vi "gen rand secenario.vi"(8 "error in (no error)":errorcluster, 10 "rand limits":T3={"# Number of emitters"=84, "# Number of frequency per emitter"={"Numeric"=0, "Numeric"=22}, "Frequency range"={"Numeric"=158778625.95419848, "Numeric"=2894656488.5496182}, "Frequency dispersion for each emitter"={"Numeric"=0.0, "Numeric"=1181732.2396298076}, "PRF range (Hz)"={"Numeric"=33.59056776941936, "Numeric"=576.0533087800792}, "Duty cycle - pulse in PRI"={"Numeric"=0.026717557251908396, "Numeric"=0.11832061068702289}, "Amplitude (dB)"={"Numeric"=-34.62595419847328, "Numeric"=-51.11450381679389}, "Modulation depth"={"Numeric"=19162.08437325717, "Numeric"=1181732.2396298076}, "CW"=TRUE, "LFM"=TRUE, "DOA (DEG)"={"Numeric"=0.0, "Numeric"=1181732.2396298076}, "start time (Sec)"=0.0, "end time (Sec)"=50.0, "BPSK"=TRUE, "QPSK"=TRUE, "ARB"=FALSE} {"DOA (DEG)" scale=0.0..360.0 scale format="%#_6f"; "Modulation depth" scale=1000.0..10000000.0 scale format="%#_6pHz"; "Amplitude (dB)" scale format="%#_6fdB"; "Duty cycle - pulse in PRI" scale=0.0..1.0 scale format="%#_6f"; "PRF range (Hz)" scale=1.0..3000.0 scale format="%#_6pHz"; "Frequency dispersion for each emitter" scale=1000000.0..100000000.0 scale format="%#_6pHz"; "Frequency range" scale=975000000.0..2225000000.0 scale format="%#_4pHz"; "# Number of frequency per emitter" scale=0.01..3000.0; "# Number of emitters" scale=0.0..200.0}, 11 "device_type in":refnum<class "device_type.lvclass">) -> (0 "error out":errorcluster, 2 "transmitters":T1[](array[typedef]) {"t end" format="%#_3p"; "t start" format="%#_3p"; "DOA" format="%#_3p"; "mod depth" format="%#_3p"}, 3 "device_type out":refnum<class "device_type.lvclass">)   [LabVIEW 2021, in "device_type.lvclass"]
uses:
  device_type.lvclass
  pulse_tx_vis/CTL/random_limits.ctl
  pulse_tx_vis/CTL/emitter params.ctl
  pulse_tx_vis/CTL/mode_type.ctl
  <vilib>/numeric/Random Number (Range) DBL.vi
  <vilib>/numeric/Random Number (Range) U64.vi
  <vilib>/numeric/sub_Random U32.vi
  device_type.lvclass/device_type.ctl
panel:
  # "modulation \ntypes:"
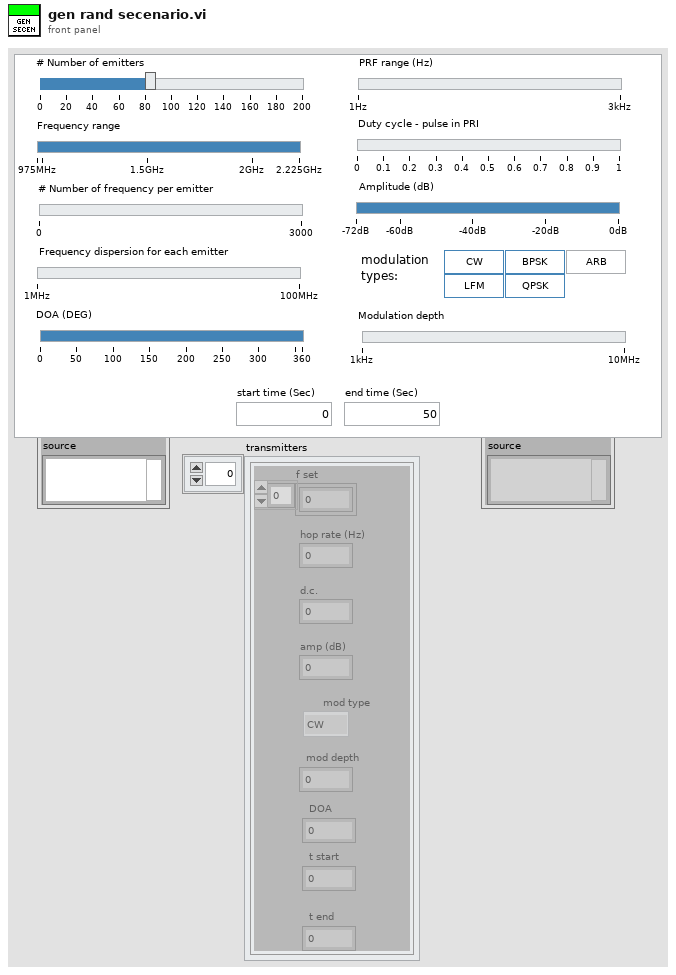
[diagram p1: front panel]
types:
  T1 = typedef "emitter params.ctl" = cluster{"f set":dbl[], "hop rate (Hz)":dbl, "d.c.":dbl, "amp (dB)":dbl, "mod type":T2, "mod depth":dbl, "DOA":dbl, "t start":dbl, "t end":dbl}
  T2 = typedef "mode_type.ctl" = enum8{"CW", "from memory 1", "NC - cw", "LFM", "BPSK", "QPSK"}
  T3 = typedef "random_limits.ctl" = cluster{"# Number of emitters":u32, "# Number of frequency per emitter":cluster{"Numeric":u32, "Numeric":u32}, "Frequency range":cluster{"Numeric":dbl, "Numeric":dbl}, "Frequency dispersion for each emitter":cluster{"Numeric":dbl, "Numeric":dbl}, "PRF range (Hz)":cluster{"Numeric":dbl, "Numeric":dbl}, "Duty cycle - pulse in PRI":cluster{"Numeric":dbl, "Numeric":dbl}, "Amplitude (dB)":cluster{"Numeric":dbl, "Numeric":dbl}, "Modulation depth":cluster{"Numeric":dbl, "Numeric":dbl}, "CW":bool, "LFM":bool, "DOA (DEG)":cluster{"Numeric":dbl, "Numeric":dbl}, "start time (Sec)":dbl, "end time (Sec)":dbl, "BPSK":bool, "QPSK":bool, "ARB":bool}
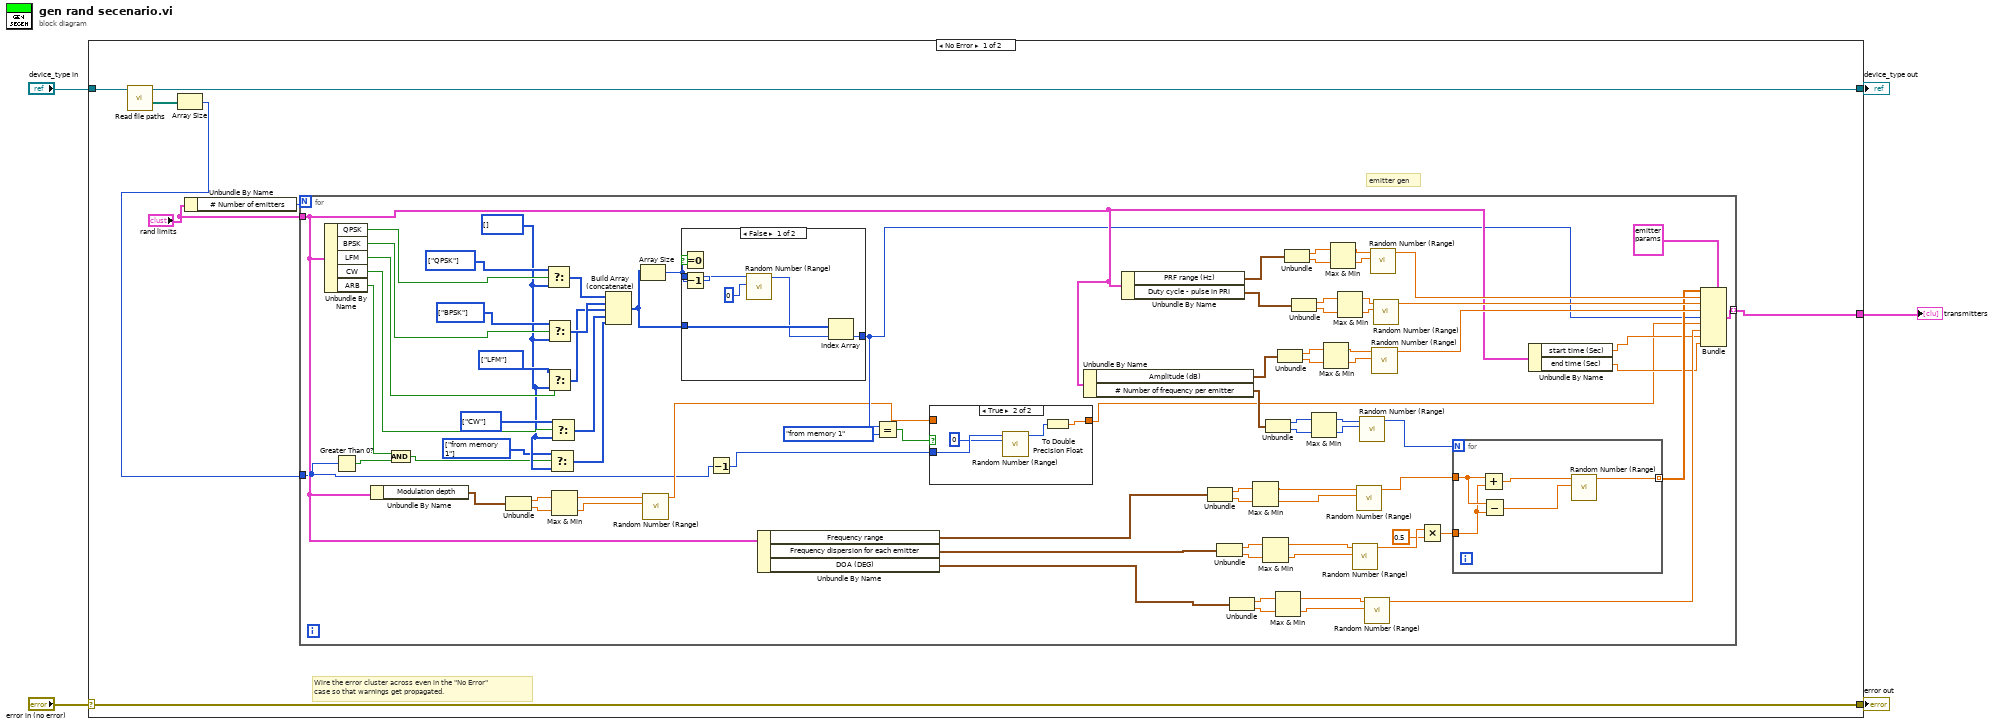
[diagram p0: block diagram]
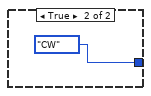
[diagram p3: hidden frame]
diagram:
  n1 = case shown="No Error" "error in (no error)" {
    selector: "error in (no error)" -> [w13 w115]
    tunnel: [w13 w115] -> w4
    tunnel: [w8 w114] -> w2
    tunnel: "device_type in" -> [w9 w114]
    tunnel: [w11 _] -> w1
    frame No Error {
      # "emitter gen"
      # "Wire the error cluster across even in the \"No Error\"\ncase so that warnings get propagated."
      n2 = call-dynamic "Read file paths.vi"("device_type in"=w9) -> ("IQ file path"=w7:path[], "device_type out"=w8:refnum<class "device_type.lvclass">)  [unwired: 7 in, 2 out]
      n3 = Array Size(array=w7) -> (size(s)=w6:i32)
      n4 = Unbundle By Name("rand limits") -> ("# Number of emitters"=w12:u32)
      n5 = for {
        N: w12 -> [_]
        tunnel: [w88] -> w11 mode=indexing
        tunnel: "rand limits" -> [w30]
        tunnel: w6 -> [w15]
        w24 = T2[] [enum."from memory 1"] items=["CW", "from memory 1", "NC - cw", "LFM", "BPSK", "QPSK"] ("t")
        w51 = T2[] [enum."QPSK"] items=["CW", "from memory 1", "NC - cw", "LFM", "BPSK", "QPSK"]
        w25 = T2[] [] items=["CW", "from memory 1", "NC - cw", "LFM", "BPSK", "QPSK"]
        w50 = T2[] [enum."BPSK"] items=["CW", "from memory 1", "NC - cw", "LFM", "BPSK", "QPSK"]
        w49 = T2[] [enum."LFM"] items=["CW", "from memory 1", "NC - cw", "LFM", "BPSK", "QPSK"]
        w48 = T2[] [enum."CW"] items=["CW", "from memory 1", "NC - cw", "LFM", "BPSK", "QPSK"]
        n6 = Unbundle By Name(w30) -> ("QPSK"=w42:bool, "BPSK"=w41:bool, "LFM"=w40:bool, "CW"=w39:bool, "ARB"=w21:bool)
        n7 = Greater Than 0?(x=w15) -> (x > 0?=w20:bool)
        n8 = Unbundle By Name(w30) -> ("Modulation depth"=w29:cluster{"Numeric":dbl, "Numeric":dbl})
        n9 = And(x=w21, y=w20) -> (x .and. y?=w19:bool)
        n10 = Unbundle(w29) -> ("Numeric"=w62:dbl, "Numeric"=w61:dbl)
        n11 = Select(t=w51, s=w42, f=w25) -> (s? t:f=w58:T2[])
        n12 = Select(t=w50, s=w41, f=w25) -> (s? t:f=w57:T2[])
        n13 = Select(t=w49, s=w40, f=w25) -> (s? t:f=w56:T2[])
        n14 = Select(t=w24, s=w19, f=w25) -> (s? t:f=w26:T2[])
        n15 = Select(t=w48, s=w39, f=w25) -> (s? t:f=w27:T2[])
        n16 = Max & Min(x=w62, y=w61) -> (max(x,y)=w60:dbl, min(x,y)=w59:dbl)
        n17 = Build Array (concatenate)(w58, w57, w56, w27, w26) -> (w55:T2[])
        n18 = Array Size(array=w55) -> (size(s)=w53:i32)
        n19 = call-poly <vilib>:"Random Number (Range).vi"("lower bound (0)"=w59, "upper bound (100)"=w60) -> ("number"=w18:dbl)  [unwired: 9 in]
        n20 = Equal To 0?(x=w53) -> (x = 0?=w54:bool)
        n21 = Decrement(x=w53) -> (x-1=w52:i32)
        n22 = case shown="False" w54 {
          tunnel: w55 -> [w106 _]
          tunnel: [w104 mode_type."CW" ("mod type")] -> w23
          tunnel: w52 -> [w103 _]
          frame False {
            n23 = call-poly <vilib>:"Random Number (Range).vi"("lower bound (0)"=u64 0, "upper bound (100)"=w103) -> ("number"=w105:u64)  [unwired: 9 in]
            n24 = Index Array(array=w106, index=w105) -> (element=w104:T2)
          }
          frame True {
          }
        }
        n25 = Decrement(x=w15) -> (x-1=w14:i32)
        n26 = Unbundle By Name(w30) -> ("Frequency range"=w28:cluster{"Numeric":dbl, "Numeric":dbl}, "Frequency dispersion for each emitter"=w33:cluster{"Numeric":dbl, "Numeric":dbl}, "DOA (DEG)"=w34:cluster{"Numeric":dbl, "Numeric":dbl})
        n27 = Equal?(x=w23, y=mode_type."from memory 1") -> (x = y?=w16:bool)
        n28 = case shown="True" w16 {
          tunnel: w18 -> [w98 _]
          tunnel: [w98 w99] -> w17
          tunnel: w14 -> [_ w102]
          frame False {
          }
          frame True {
            n29 = call-poly <vilib>:"Random Number (Range).vi"("lower bound (0)"=u64 0, "upper bound (100)"=w102) -> ("number"=w100:u64)  [unwired: 9 in]
            n30 = To Double Precision Float(number=w100) -> (double precision float=w99:dbl)
          }
        }
        n31 = Unbundle By Name(w30) -> ("Amplitude (dB)"=w36:cluster{"Numeric":dbl, "Numeric":dbl}, "# Number of frequency per emitter"=w35:cluster{"Numeric":u32, "Numeric":u32})
        n32 = Unbundle By Name(w30) -> ("PRF range (Hz)"=w38:cluster{"Numeric":dbl, "Numeric":dbl}, "Duty cycle - pulse in PRI"=w37:cluster{"Numeric":dbl, "Numeric":dbl})
        n33 = Unbundle(w28) -> ("Numeric"=w70:dbl, "Numeric"=w69:dbl)
        n34 = Unbundle(w33) -> ("Numeric"=w65:dbl, "Numeric"=w66:dbl)
        n35 = Unbundle(w34) -> ("Numeric"=w45:dbl, "Numeric"=w44:dbl)
        n36 = Max & Min(x=w70, y=w69) -> (max(x,y)=w68:dbl, min(x,y)=w67:dbl)
        n37 = Max & Min(x=w65, y=w66) -> (max(x,y)=w64:dbl, min(x,y)=w63:dbl)
        n38 = Unbundle(w35) -> ("Numeric"=w73:u32, "Numeric"=w74:u32)
        n39 = Max & Min(x=w45, y=w44) -> (max(x,y)=w46:dbl, min(x,y)=w47:dbl)
        n40 = Unbundle(w36) -> ("Numeric"=w84:dbl, "Numeric"=w83:dbl)
        n41 = Unbundle(w38) -> ("Numeric"=w78:dbl, "Numeric"=w77:dbl)
        n42 = Unbundle(w37) -> ("Numeric"=w81:dbl, "Numeric"=w82:dbl)
        n43 = Max & Min(x=w73, y=w74) -> (max(x,y)=w72:u32, min(x,y)=w71:u32)
        n44 = Max & Min(x=w84, y=w83) -> (max(x,y)=w86:dbl, min(x,y)=w85:dbl)
        n45 = Max & Min(x=w78, y=w77) -> (max(x,y)=w76:dbl, min(x,y)=w75:dbl)
        n46 = Max & Min(x=w81, y=w82) -> (max(x,y)=w80:dbl, min(x,y)=w79:dbl)
        n47 = call-poly <vilib>:"Random Number (Range).vi"("lower bound (0)"=w63, "upper bound (100)"=w64) -> ("number"=w93:dbl)  [unwired: 9 in]
        n48 = call-poly <vilib>:"Random Number (Range).vi"("lower bound (0)"=w67, "upper bound (100)"=w68) -> ("number"=w91:dbl)  [unwired: 9 in]
        n49 = call-poly <vilib>:"Random Number (Range).vi"("lower bound (0)"=w71, "upper bound (100)"=w72) -> ("number"=w87:u64)  [unwired: 9 in]
        n50 = call-poly <vilib>:"Random Number (Range).vi"("lower bound (0)"=w47, "upper bound (100)"=w46) -> ("number"=w43:dbl)  [unwired: 9 in]
        n51 = call-poly <vilib>:"Random Number (Range).vi"("lower bound (0)"=w75, "upper bound (100)"=w76) -> ("number"=w96:dbl)  [unwired: 9 in]
        n52 = call-poly <vilib>:"Random Number (Range).vi"("lower bound (0)"=w85, "upper bound (100)"=w86) -> ("number"=w94:dbl)  [unwired: 9 in]
        n53 = call-poly <vilib>:"Random Number (Range).vi"("lower bound (0)"=w79, "upper bound (100)"=w80) -> ("number"=w95:dbl)  [unwired: 9 in]
        n54 = Multiply(x=w93, y=0.5) -> (x*y=w90:dbl)
        n55 = for {
          N: w87 -> [_]
          tunnel: w91 -> [w113]
          tunnel: w90 -> [w112]
          tunnel: [w109] -> w89 mode=indexing
          n56 = Add(x=w113, y=w112) -> (x+y=w110:dbl)
          n57 = Subtract(x=w113, y=w112) -> (x-y=w111:dbl)
          n58 = call-poly <vilib>:"Random Number (Range).vi"("lower bound (0)"=w111, "upper bound (100)"=w110) -> ("number"=w109:dbl)  [unwired: 9 in]
        }
        n59 = Unbundle By Name(w30) -> ("start time (Sec)"=w32:dbl, "end time (Sec)"=w31:dbl)
        n60 = Bundle(cluster=T1 {"f set"=[1000000.0], "hop rate (Hz)"=300000.0, "d.c."=0.0, "amp (dB)"=-20.0, "mod type"=enum."CW", "mod depth"=0.0, "DOA"=0.0, "t start"=0.0, "t end"=0.0} ("Cluster"), "f set"=w89, "hop rate (Hz)"=w96, "d.c."=w95, "amp (dB)"=w94, "mod type"=w23, "mod depth"=w17, "DOA"=w43, "t start"=w32, "t end"=w31) -> (w88:T1)
      }
    }
    frame Error {
    }
  }
  "error out" <- w4
  "device_type out" <- w2
  "transmitters" <- w1
